vi "Subpanel_SectionA1.vi"() -> ()   [LabVIEW 2016]
doc: "einfaches Template für Consumer/Producer Design (User). \n\n9.12.13 / sige"
uses:
  Message Queue/private/MessageQueue.MessageTypeDef.ctl
  <vilib>/Utility/error.llb/Error Cluster From Error Code.vi
  <vilib>/ErrorRing/Error Ring.xnode
panel:
  in  "Stop Button":bool
  in  "Command":bool
  in  "Data":dbl
  # "A1"
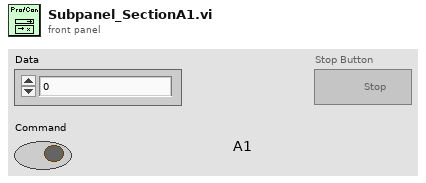
[diagram p1: front panel]
types:
  T1 = typedef "MessageQueue.MessageTypeDef.ctl" = cluster{"Message":string, "Data":variant}
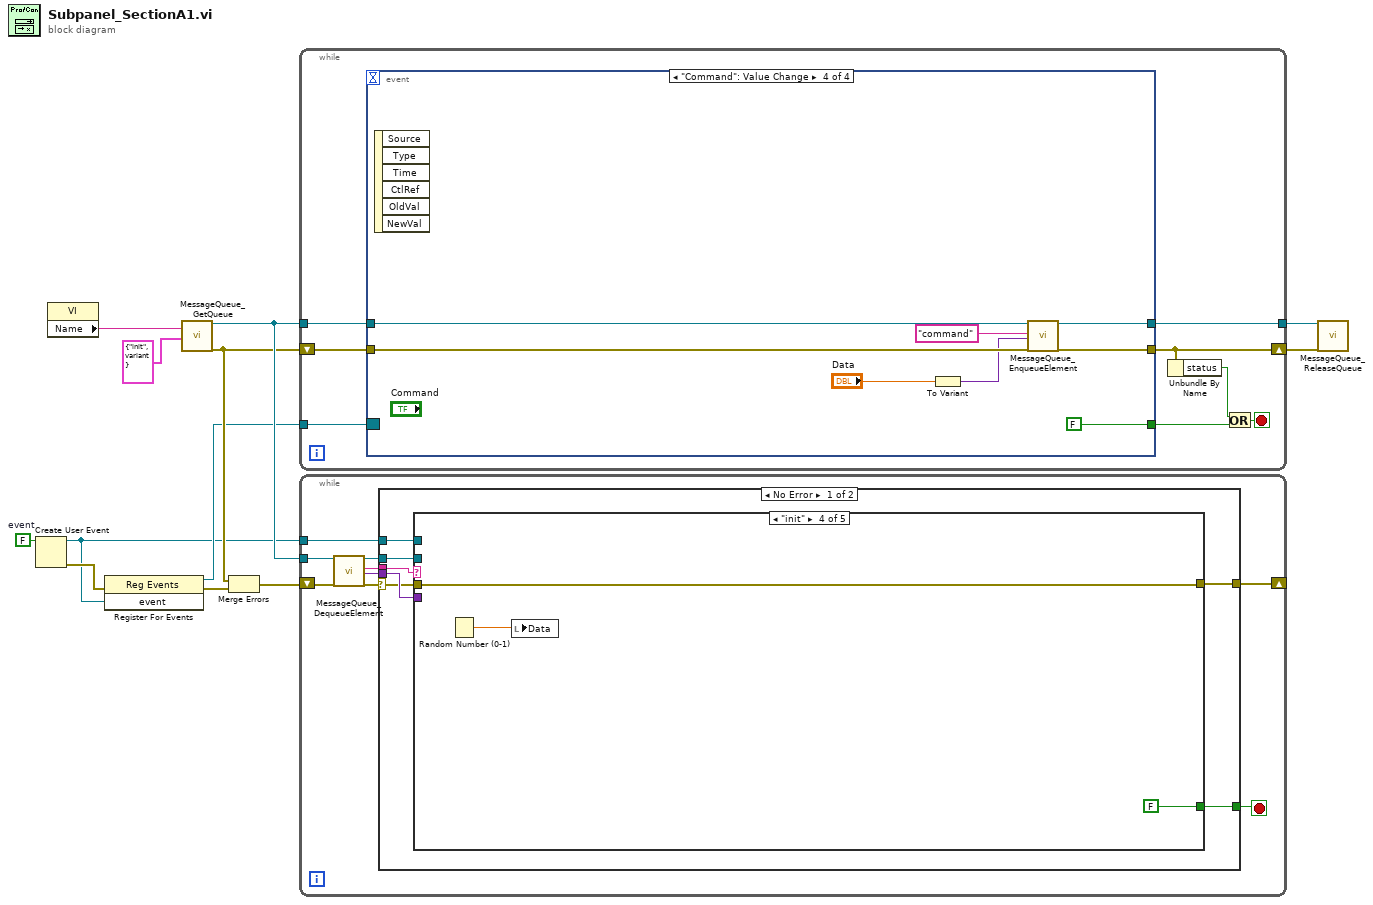
[diagram p0: block diagram]
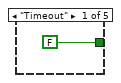
[diagram p2: hidden frame]
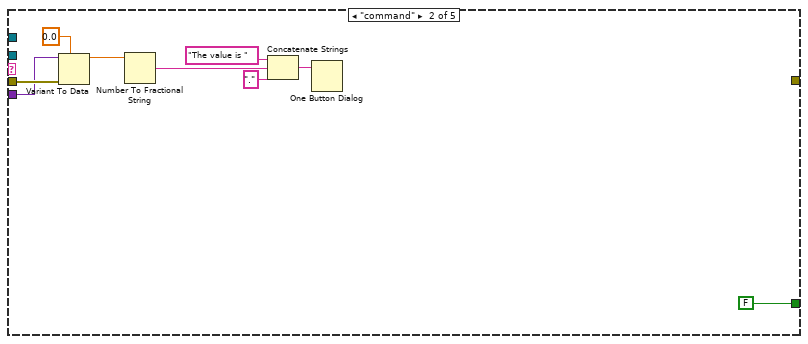
[diagram p3: hidden frame]
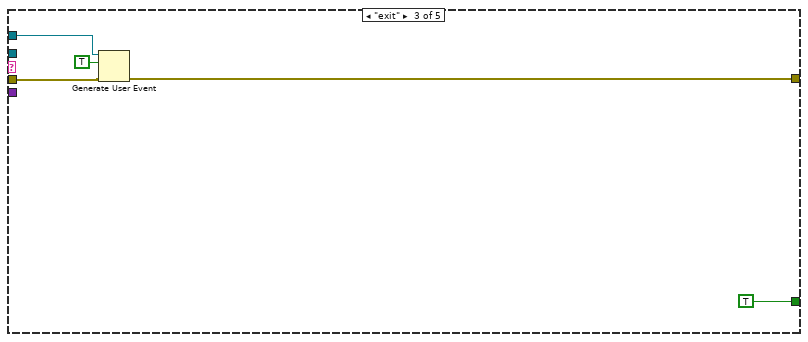
[diagram p4: hidden frame]
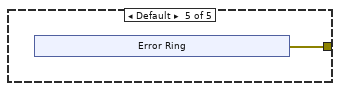
[diagram p5: hidden frame]
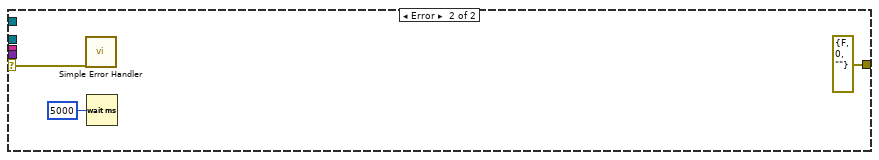
[diagram p6: hidden frame]
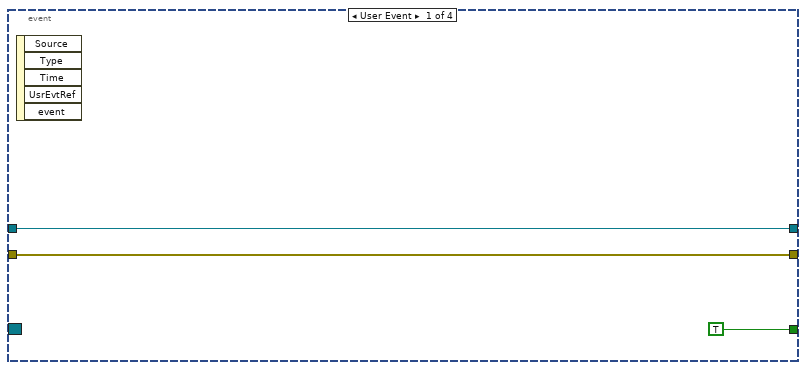
[diagram p7: hidden frame]
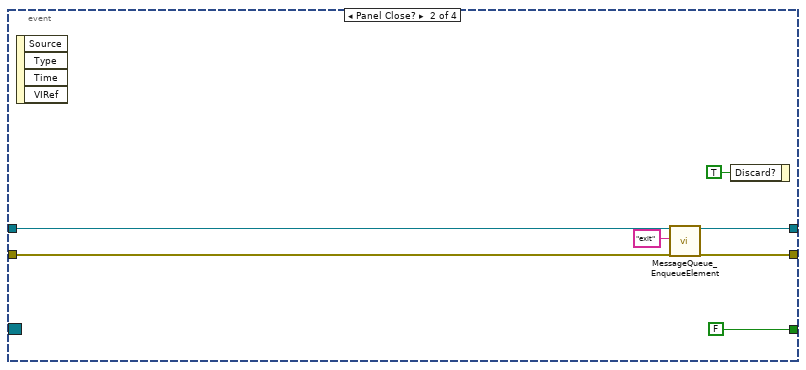
[diagram p8: hidden frame]
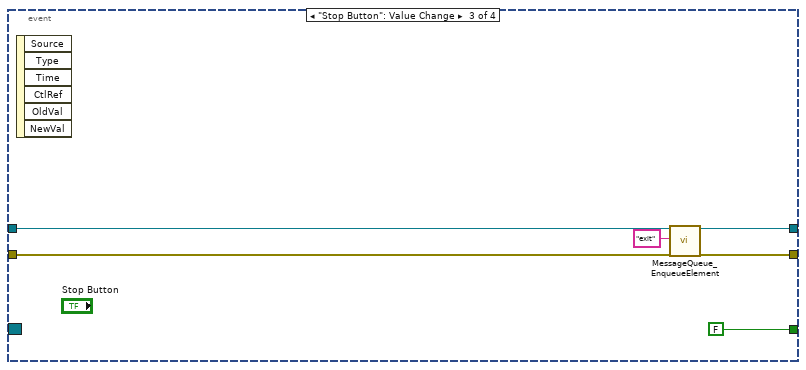
[diagram p9: hidden frame]
diagram:
  w4 = FALSE  # event
  n1 = Create User Event(user event datatype=w4) -> (user event=w2:refnum<user-event>, error out=w3:errorcluster)  [unwired: 1 in]
  n2 = property class="VI"() -> ("Name"=w1:string)  [unwired: 2 in, 2 out]
  n3 = register-events(error in=w3, w2) -> (reference out=w6:refnum<event-registration>, error out=w8:errorcluster)  [unwired: 1 in]
  n4 = call "MessageQueue_GetQueue.vi"("Name"=w1, "OptionalInitValue"=T1 {"Message"="init", "Data"=variant}) -> ("QueueOut"=w10:refnum<queue>, "ErrorOut"=w7:errorcluster)  [unwired: 15 in, 1 out]
  n5 = Merge Errors(w7, w8) -> (w5:errorcluster)
  n6 = while {
    tunnel: w10 -> [w20]
    tunnel: [w19] -> w12
    shift-right: [w16] -> w11
    shift-left: w7 -> [w18]
    tunnel: w6 -> [w13]
    stop <- w15 stop-if-true
    n7 = event shown="[3] \"Command\": Value Change" {
      selector: w13 -> [_ _ _ _]
      dyn-events: _ -> [_ _ _ _]
      timeout: _ -> [_ _ _ _]
      tunnel: w20 -> [w22 w30 w36 w44]
      tunnel: [w22 w29 w35 w43] -> w19
      tunnel: [w21 w28 w34 w42] -> w16
      tunnel: w18 -> [w21 w27 w33 w41]
      tunnel: [TRUE FALSE FALSE FALSE] -> w17
      event User Event {
        n8 = event-data() -> ()  [unwired: 1 in, 5 out]
      }
      event Panel Close? {
        n9 = event-data() -> ()  [unwired: 1 in, 4 out]
        n10 = call "MessageQueue_EnqueueElement.vi"("QueueIn"=w30, "Message"="exit", "ErrorIn"=w27) -> ("QueueOut"=w29:refnum<queue>, "ErrorOut"=w28:errorcluster)  [unwired: 15 in]
        n11 = event-data("Discard?"=TRUE) -> ()  [unwired: 1 in, 1 out]
      }
      event "Stop Button": Value Change {
        n12 = event-data() -> ()  [unwired: 1 in, 6 out]
        n13 = call "MessageQueue_EnqueueElement.vi"("QueueIn"=w36, "Message"="exit", "ErrorIn"=w33) -> ("QueueOut"=w35:refnum<queue>, "ErrorOut"=w34:errorcluster)  [unwired: 15 in]
      }
      event "Command": Value Change {
        n14 = event-data() -> ()  [unwired: 1 in, 6 out]
        n15 = To Variant(anything="Data") -> (Variant=w37:variant)
        n16 = call "MessageQueue_EnqueueElement.vi"("QueueIn"=w44, "Message"="command", "Data"=w37, "ErrorIn"=w41) -> ("QueueOut"=w43:refnum<queue>, "ErrorOut"=w42:errorcluster)  [unwired: 14 in]
      }
    }
    n17 = Unbundle By Name(w16) -> ("status"=w14:bool)
    n18 = Or(x=w14, y=w17) -> (x .or. y?=w15:bool)
  }
  n19 = while {
    tunnel: w10 -> [w53]
    tunnel: w2 -> [w46]
    shift-right: [w45] -> _
    shift-left: w5 -> [w47]
    stop <- w48 stop-if-true
    n20 = call "MessageQueue_DequeueElement.vi"("QueueIn"=w53, "ErrorIn"=w47) -> ("QueueOut"=w51:refnum<queue>, "Message"=w50:string, "Data"=w49:variant, "ErrorOut"=w52:errorcluster)  [unwired: 13 in, 1 out]
    n21 = case shown="No Error" w52 {
      selector: w52 -> [w56 w87]
      tunnel: w51 -> [w60 _]
      tunnel: w50 -> [w59 _]
      tunnel: w49 -> [w58 _]
      tunnel: [w57 _] -> w48
      tunnel: w46 -> [w55 _]
      tunnel: [w54 errorcluster {"status"=FALSE, "code"=0, "source"=""} ("error out")] -> w45
      frame No Error {
        n22 = case shown="\"init\"" w59 {
          tunnel: w60 -> [_ _ _ _ _]
          tunnel: w58 -> [_ w67 _ _ _]
          tunnel: [FALSE FALSE TRUE FALSE _] -> w57
          tunnel: w56 -> [_ w69 w73 w76 _]
          tunnel: w55 -> [_ _ w72 _ _]
          tunnel: [_ _ w71 w76 w79] -> w54
          frame "Timeout" {
          }
          frame "command" {
            n23 = Variant To Data(error in=w69, type=0.0 ("Data"), Variant=w67) -> (data=w66:dbl)  [unwired: 1 out]
            n24 = Number To Fractional String(number=w66) -> (F-format string=w63:string)  [unwired: 3 in]
            n25 = Concatenate Strings("The value is " ("string"), w63, "." ("string")) -> (w62:string)
            n26 = One Button Dialog(message=w62) -> ()  [unwired: 1 in, 1 out]
          }
          frame "exit" {
            n27 = Generate User Event(user event=w72, event data cluster=TRUE ("event data"), error in=w73) -> (error out=w71:errorcluster)  [unwired: 1 in, 1 out]
          }
          frame "init" {
            n28 = Random Number (0-1)() -> (number: 0 to 1=w77:dbl)
            n29 = local write "Data"(w77) -> ()
          }
          frame Default {
            n30 = xnode "Error Ring"() -> ("error out"=w79:errorcluster)
          }
        }
      }
      frame Error {
        n31 = call <vilib>:"Simple Error Handler.vi"("error in (no error)"=w87) -> ()  [unwired: 4 in, 5 out]
        n32 = Wait (ms)(milliseconds to wait=u32 5000) -> ()  [unwired: 1 out]
      }
    }
  }
  n33 = call "MessageQueue_ReleaseQueue.vi"("QueueIn"=w12, "ErrorIn"=w11) -> ()  [unwired: 15 in, 3 out]
